vi "whole.vi"() -> ()   [LabVIEW 2017]
panel:
  out "error out":errorcluster
  in  "Reste IP":string="192.168.10.17"
  in  "TDC IP":string[](array[string])=["192.168.10.20", "192.168.10.22"]
  in  "Calib":bool
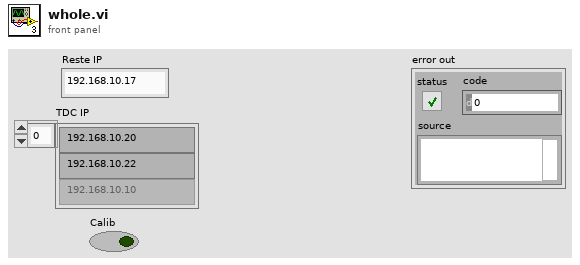
[diagram p1: front panel]
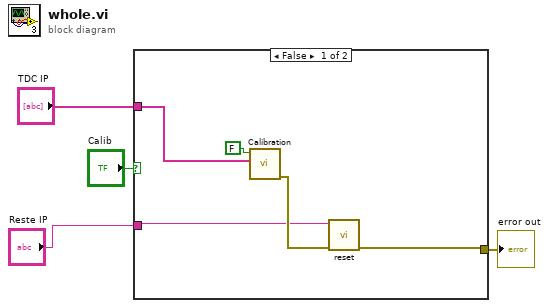
[diagram p0: block diagram]
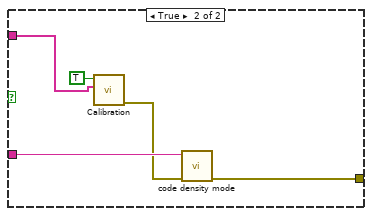
[diagram p2: hidden frame]
diagram:
  n1 = case shown="False" "Calib" {
    tunnel: "TDC IP" -> [w8 w13]
    tunnel: "Reste IP" -> [w5 w12]
    tunnel: [w6 w10] -> w1
    frame False {
      n2 = call "Calibration.vi"("Array 2"=w8, "SMA mode"=FALSE) -> ("error out"=w7:errorcluster)  [unwired: 9 in]
      n3 = call "reset.vi"("error in (no error)"=w7, "IP address"=w5) -> ("error out"=w6:errorcluster)  [unwired: 9 in]
    }
    frame True {
      n4 = call "Calibration.vi"("Array 2"=w13, "SMA mode"=TRUE) -> ("error out"=w11:errorcluster)  [unwired: 9 in]
      n5 = call "code density mode.vi"("error in (no error)"=w11, "IP address"=w12) -> ("error out"=w10:errorcluster)  [unwired: 9 in]
    }
  }
  "error out" <- w1
